vi "Reset.vi"(8 "error in (no error)":errorcluster, 11 "Sequence in":refnum<class "Sequence.lvclass">) -> (0 "error out":errorcluster, 3 "Sequence out":refnum<class "Sequence.lvclass">)   [LabVIEW 2019, in "Sequence.lvclass"]
uses:
  Sequence.lvclass
  Sequence.lvclass/Sequence.ctl
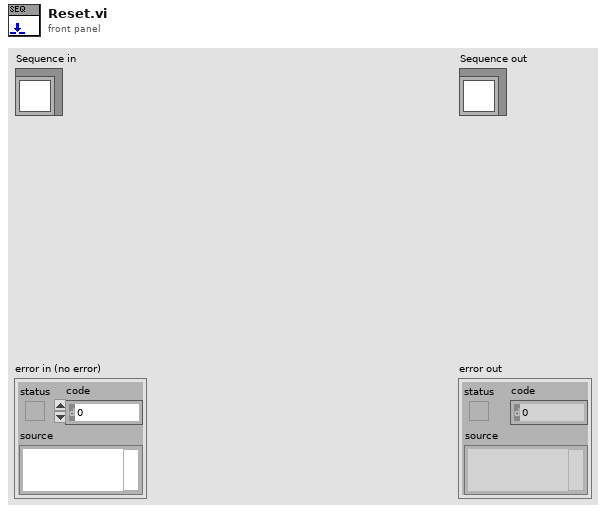
[diagram p1: front panel]
types:
  T1 = typedef "mWaveTestStep.ctl" = cluster{"StepType":T2, "RF In/Out":T3, "Module/Raster":i32, "Polarization":T4, "AO-64 Array":dbl[], "Position":T5[]}
  T2 = typedef "TestStepTypes.ctl" = enum16{"MotionFF-M2", "Motion", "SweepTest", "RasterTest", "Finish", "64ModuleCfg"}
  T3 = typedef "RF Direction.ctl" = enum16{"Tx - RF In", "Rx - RF Out"}
  T4 = typedef "PolarizationSelect.ctl" = enum16{"Vertical", "Horizontal"}
  T5 = typedef "singleAxisMoveDef.ctl" = cluster{"mmWave Axis":T6, "eng. value":dbl}
  T6 = typedef "mmWaveAxis.ctl" = string
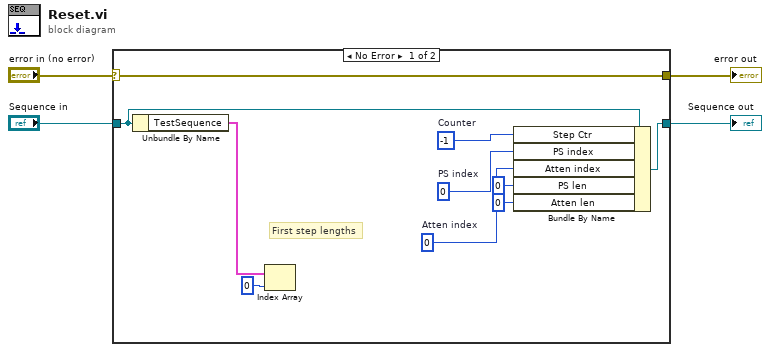
[diagram p0: block diagram]
diagram:
  n1 = case shown="No Error" "error in (no error)" {
    selector: "error in (no error)" -> [w14 w16]
    tunnel: [w14 w16] -> w3
    tunnel: [w13 w15] -> w1
    tunnel: "Sequence in" -> [w9 w15]
    frame No Error {
      w10 = 0  # Atten index
      w11 = 0  # PS index
      w12 = -1  # Counter
      # "First step lengths"
      n2 = Unbundle By Name(w9) -> ("TestSequence"=w8:T1[])
      n3 = Index Array(array=w8, index=0) -> ()  [unwired: 1 out]
      n4 = Bundle By Name(cluster=w9, "Step Ctr"=w12, "PS index"=w11, "Atten index"=w10, "PS len"=0 ("Execution.PS len"), "Atten len"=0 ("Execution.Atten len")) -> (w13:refnum<class "Sequence.lvclass">)
    }
    frame Error {
    }
  }
  "error out" <- w3
  "Sequence out" <- w1
